vi "Runner.FilterDefineTest.vi"(10 "Paths":path[](array[path])) -> (2 "Filtered Paths":path[](array[path]))   [LabVIEW 2013, in "Caraya.lvlib" / "Test Runner.lvclass"]
uses:
  Test Runner.lvclass
  Test/Define Test.vi
  Test/Test.lvclass
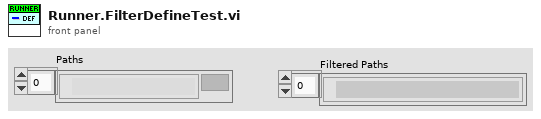
[diagram p1: front panel]
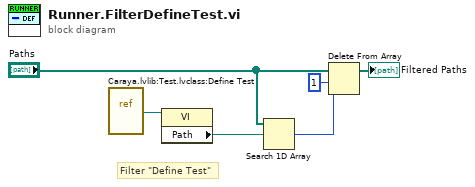
[diagram p0: block diagram]
diagram:
  # "Filter \"Define Test\""
  n1 = vi-ref "Caraya.lvlib:Test.lvclass:Define Test.vi"() -> (w3:refnum<vi>)
  n2 = property class="VI"(reference=w3) -> ("Path"=w6:path)  [unwired: 1 in, 2 out]
  n3 = Search 1D Array(1D array="Paths", element=w6) -> (index of element=w5:i32)  [unwired: 1 in]
  n4 = Delete From Array(array="Paths", length=1, index=w5) -> (array with subset deleted=→"Filtered Paths":path[])  [unwired: 1 out]
